vi "play-AFM-CS-imaging-dirty.vi"() -> ()   [LabVIEW 2017]
uses:
  raster-scan-params.ctl
  controls/PI-params.ctl
  controls/boolean_info.ctl
  <vilib>/userdefined/High Color/nirio_resource_hc.ctl
  <vilib>/Utility/file.llb/Read Delimited Spreadsheet (DBL).vi
  <vilib>/FPGAPlugInAG/cRIO-9082/niLvFpga_Open_cRIO-9082.vi
  <vilib>/rvi/interface/common/dynamic/niFpgaDynamicAddResources.vi
  <vilib>/FPGAPlugInAG/Dynamic/niLvFpga_Reset_Dynamic.vi
  <vilib>/rvi/interface/common/niFpgaWaitOnOcc.vi
  <vilib>/Utility/error.llb/Error Cluster From Error Code.vi
  <vilib>/rvi/errors/niLvFpgaAdjustHostInterfaceError.vi
  <vilib>/FPGAPlugInAG/Dynamic/niLvFpga_Run_Dynamic.vi
  <vilib>/Utility/file.llb/Write Delimited Spreadsheet (DBL).vi
  <vilib>/FPGAPlugInAG/Dynamic/niLvFpga_Close_Dynamic.vi
  <vilib>/rvi/interface/nirviOpenFPGA/nirviOpenFPGA.xnode
  FPGA Bitfiles/afmimagingcontro_FPGATargetSPARTA_cs-scanning_gCu814jKz54.lvbitx
  <vilib>/rvi/interface/nirviMethod/nirviMethod.xnode
  <vilib>/rvi/interface/nirviReadWriteControl/nirviReadWriteControl.xnode
  <vilib>/rvi/interface/nirviCloseFPGA/nirviCloseFPGA.xnode
  <vilib>/FPGAPlugInAG/Dynamic/niLvFpga_ConfigureFifo_Dynamic.vi
  <vilib>/rvi/errors/niLvFpgaMergeErrorWithErrorCode.vi
  <vilib>/rvi/interface/Simulation/niFpgaSimulationCallBeginRW.vi
  <vilib>/FPGAPlugInAG/Dynamic/niLvFpga_ReadFifo_Dynamic.vi
  NiFpgaLv.dll
  <vilib>/FPGAPlugInAG/Dynamic/niLvFpga_WriteFifo_Dynamic.vi
panel:
  in  "Z-settled-samples threshold":i16
  in  "Z-error-threshold":sgl
  out "case-selected":i16
  out "number-settled-samples-y":i16
  out "number-settled-samples-x":i16
  in  "settled-samples threshold":i16=200
  in  "error-threshold":sgl=0.1
  out "Array":i32[][](array[numeric])
  in  "zup-N":i16=5000
  out "z-control":dbl[](graph)
  out "x-axis 2":dbl[](graph)
  out "z-error":dbl[](graph)
  out "y-axis 2":dbl[](graph)
  out "size(s) 2":i32[](array[numeric])
  in  "numEntities":i16
  out "uz-":dbl[](graph)
  out "y-axis":dbl[](graph)
  out "x-axis":dbl[](graph)
  in  "z-bound":sgl=5.0
  in  "Ki-xy":sgl=0.005
  out "boolean errors":T1
  in  "raster-scan-params":T2={"TsTicks"=1600, "Stop"=TRUE, "TOL"=0.3, "ramp-rate"=-5e-06, "z-u-max"=5.0, "PI-params"={"Ki"=0.001, "setpoint"=0.0}} {"ramp-rate" format="%#_4g"; "TOL" format="%#_13g"}
  out "e(0) (threshhold init)":fxp<+/-,16,5>
  in  "STOP":bool
  out "nsamps":i32
  in  "trigger-0":bool
  in  "init Z up":sgl step=1
  in  "z_UP (case 3)":fxp<+/-,16,5>=1.0
  out "ADC-zaxis":sgl
  out "elements left":i32=1
  in  "reference traj path":path=path "C:/Users/arnold/Documents/labview/afm_imaging/data/data-in.csv"
  in  "outputData BOTH":path=path "C:/Users/arnold/Documents/labview/afm_imaging/data/data-out.csv"
  out "y iter":i32
  out "size(s)":i32
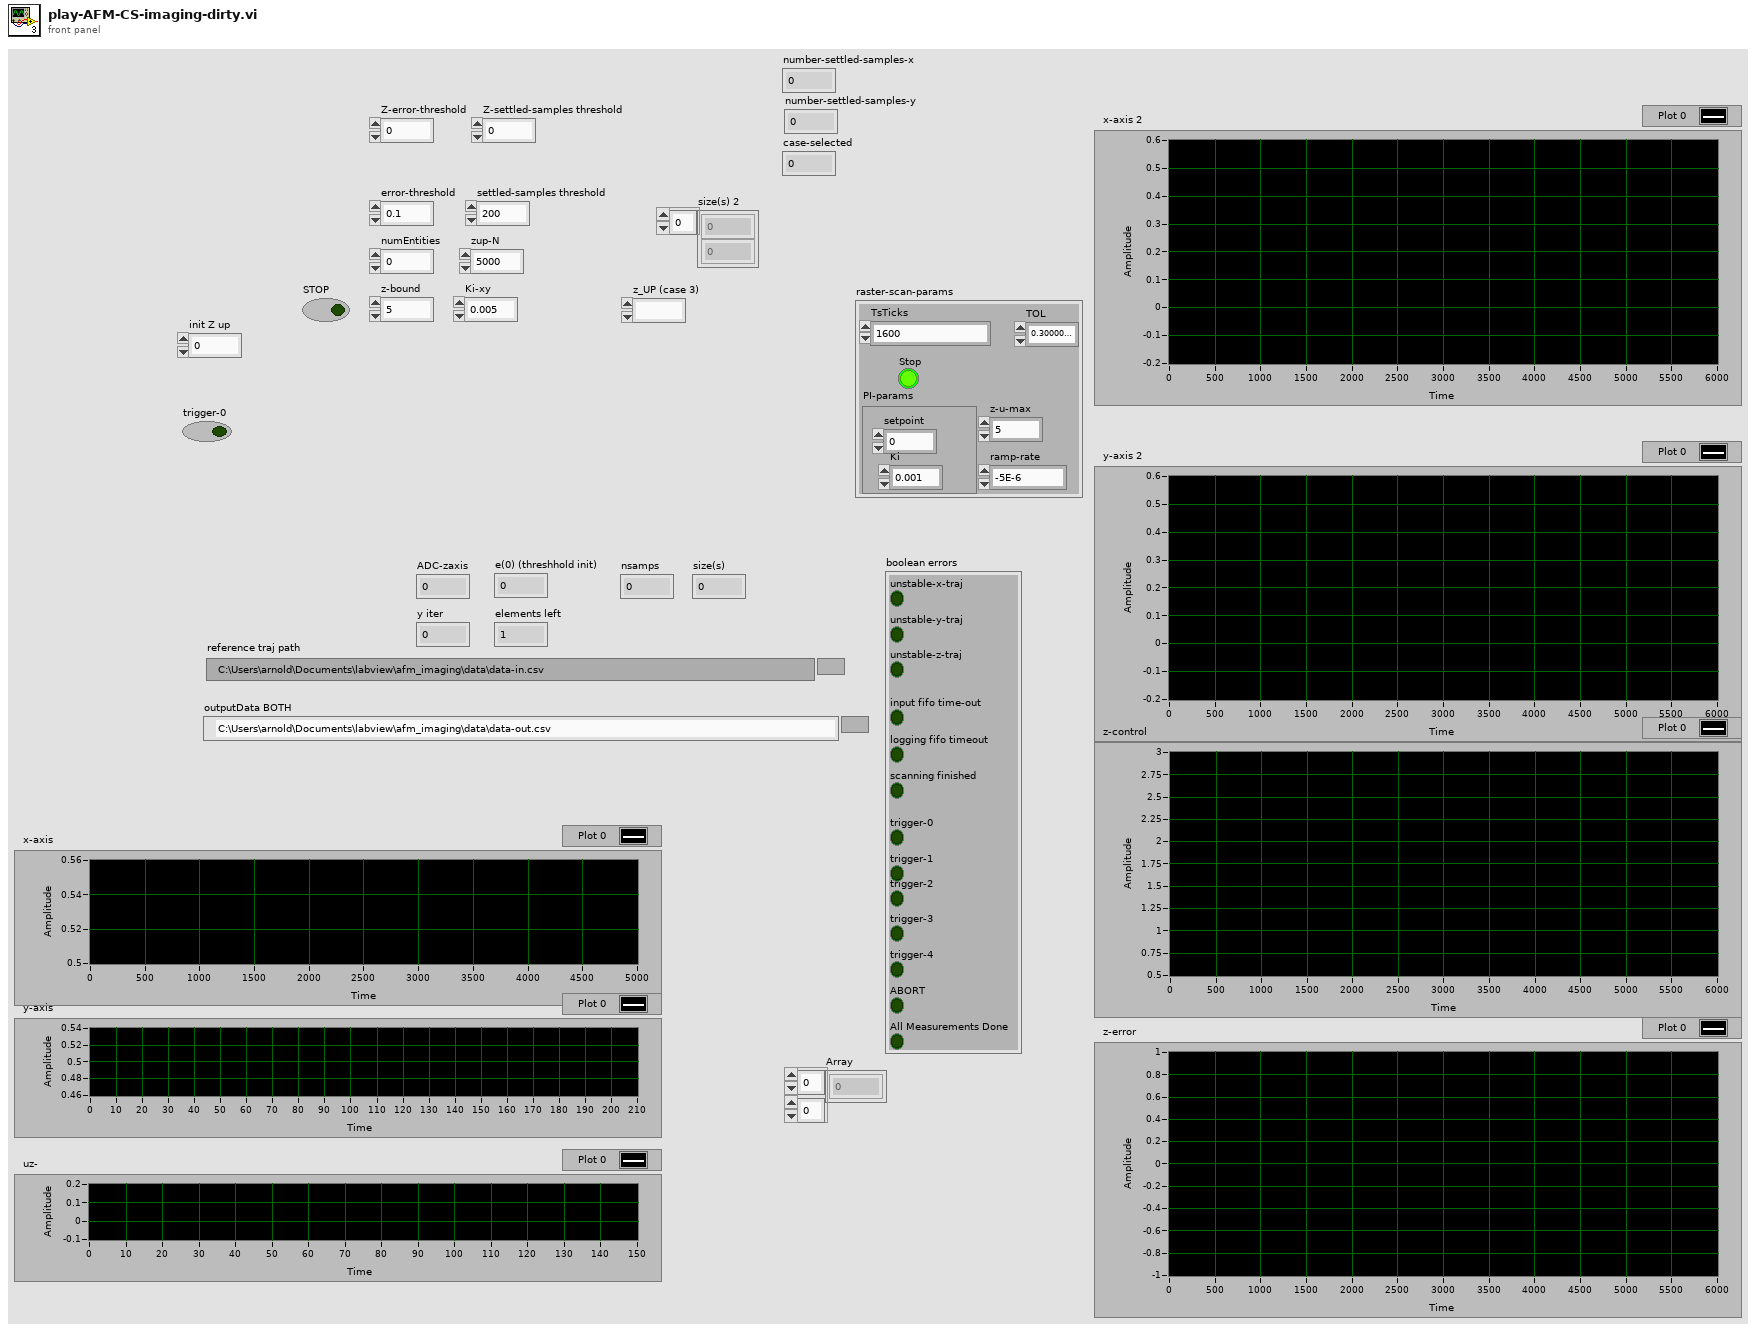
[diagram p1: front panel]
types:
  T1 = typedef "boolean_info.ctl" = cluster{"unstable-z-traj":bool, "input fifo time-out":bool, "logging fifo timeout":bool, "scanning finished":bool, "trigger-1":bool, "trigger-0":bool, "trigger-2":bool, "trigger-3":bool, "trigger-4":bool, "unstable-x-traj":bool, "unstable-y-traj":bool, "ABORT":bool, "All Measurements Done":bool}
  T2 = typedef "raster-scan-params.ctl" = cluster{"TsTicks":u32, "Stop":bool, "TOL":sgl, "ramp-rate":sgl, "z-u-max":sgl, "PI-params":T3}
  T3 = typedef "PI-params.ctl" = cluster{"Ki":sgl, "setpoint":sgl}
  T4 = typedef "nirio_resource_hc.ctl" = tag
  T5 = cluster{"unstable-z-traj":bool, "input fifo time-out":bool, "logging fifo timeout":bool, "scanning finished":bool, "trigger-1":bool, "trigger-0":bool, "trigger-2":bool, "trigger-3":bool, "trigger-4":bool, "unstable-x-traj":bool, "unstable-y-traj":bool, "ABORT":bool, "All Measurements Done":bool}
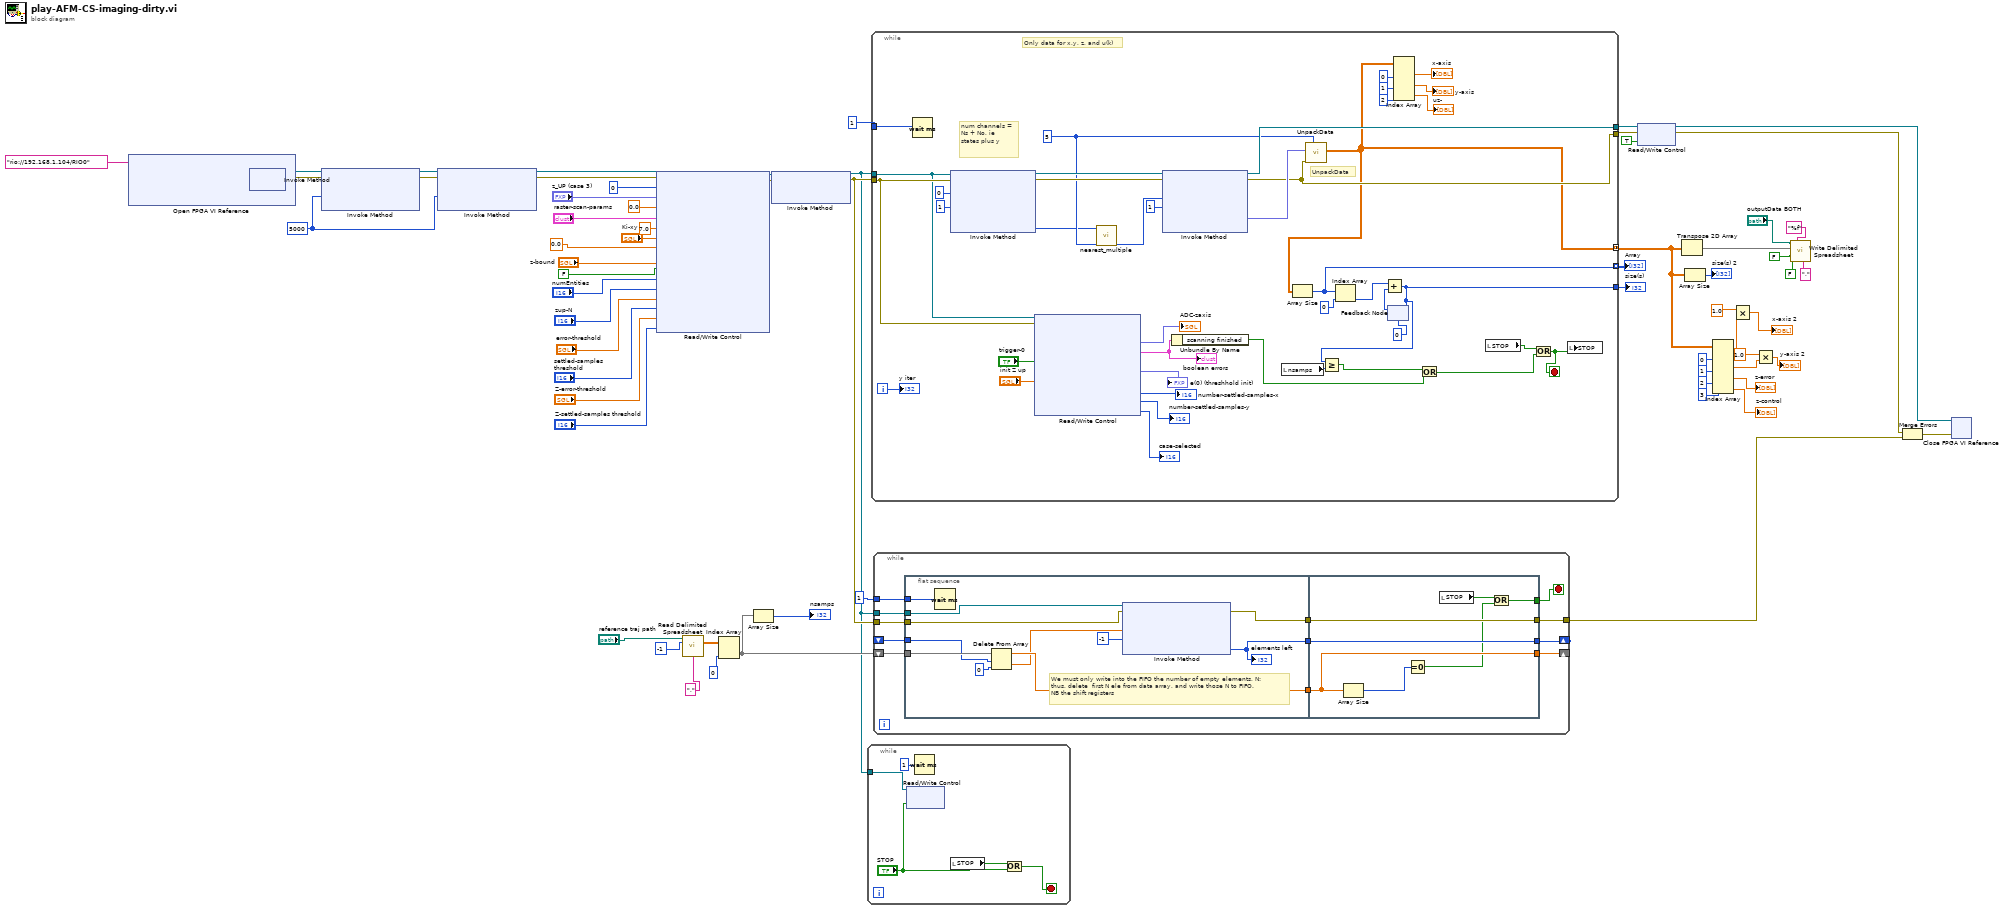
[diagram p0: block diagram]
diagram:
  w63 = 5000
  n1 = xnode "Open FPGA VI Reference"("resource name"=T4 "rio://192.168.1.104/RIO0") -> ("FPGA VI Reference Out"=w62:refnum<k20>, "error out"=w61:errorcluster)  [unwired: 1 in]
  n2 = xnode "Invoke Method"("FPGA VI Reference In"=w62, "error in"=w61) -> ("FPGA VI Reference Out"=w50:refnum<k20>, "error out"=w49:errorcluster)
  n3 = xnode "Invoke Method"("FPGA VI Reference In"=w50, "error in"=w49, "Requested Depth"=w63) -> ("FPGA VI Reference Out"=w54:refnum<k20>, "error out"=w55:errorcluster)  [unwired: 1 out]
  n4 = xnode "Invoke Method"("FPGA VI Reference In"=w54, "error in"=w55, "Requested Depth"=w63) -> ("FPGA VI Reference Out"=w65:refnum<k20>, "error out"=w64:errorcluster)  [unwired: 1 out]
  n5 = xnode "Read/Write Control"("FPGA VI Reference In"=w65, "error in"=w64, "initial case"=i16 0, "z_UP"="z_UP (case 3)", "u_z(0)"=sgl 0.0 ("u(0)"), "raster-scan-params"="raster-scan-params", "xy-bound"=sgl 7.0, "Ki-xy"="Ki-xy", "init Z up"=sgl 0.0 ("u(0)"), "z-bound"="z-bound", "trigger-0"=FALSE, "numEntities"="numEntities", "zup-N"="zup-N", "error-threshold"="error-threshold", "settled-samples threshold"="settled-samples threshold", "Z-error-threshold"="Z-error-threshold", "Z-settled-samples threshold"="Z-settled-samples threshold") -> ("FPGA VI Reference Out"=w52:refnum<k20>, "error out"=w51:errorcluster)
  n6 = call-poly <vilib>:"Read Delimited Spreadsheet.vi"("file path (dialog if empty)"="reference traj path", "number of rows (all:-1)"=-1, "delimiter (\\t)"=",") -> ("all rows"=w40:dbl[][])  [unwired: 7 in, 5 out]
  n7 = Index Array(array=w40, index (col)=0 ("dimension size")) -> (element=w47:dbl[])  [unwired: 1 in]
  n8 = Array Size(array=w47) -> (size(s)=→"nsamps":i32)
  n9 = xnode "Invoke Method"("FPGA VI Reference In"=w52, "error in"=w51) -> ("FPGA VI Reference Out"=w12:refnum<k20>, "error out"=w56:errorcluster)  [unwired: 1 in]
  n10 = while {
    tunnel: w12 -> [w72]
    stop <- w68 stop-if-true
    n11 = xnode "Read/Write Control"("FPGA VI Reference In"=w72, "ABORT"="STOP") -> ()  [unwired: 1 in, 2 out]
    n12 = Wait (ms)(milliseconds to wait=u32 1) -> ()  [unwired: 1 out]
    n13 = local read "STOP"() -> (w69:bool)
    n14 = Or(x=w69, y="STOP") -> (x .or. y?=w68:bool)
  }
  n15 = while {
    tunnel: 1 -> [w114]
    tunnel: w12 -> [w100]
    tunnel: w56 -> [w101]
    tunnel: [w107] -> w33
    tunnel: [w85] -> w16 mode=concatenating
    tunnel: [w98] -> w66
    tunnel: [w86] -> w32
    tunnel: [w76] -> w11 mode=indexing
    i -> [w99]
    stop <- w77 stop-if-true
    w91 = u32 5 ("y")
    # "num channels = Ns + No, ie states plus y"
    # "Only data for x,y, z, and u(k)"
    # "UnpackData"
    n16 = Wait (ms)(milliseconds to wait=w114) -> ()  [unwired: 1 out]
    n17 = xnode "Invoke Method"("FPGA VI Reference In"=w100, "error in"=w101, "Number of Elements"=0 ("Timeout (ms)"), "Timeout (ms)"=1) -> ("FPGA VI Reference Out"=w110:refnum<k20>, "error out"=w111:errorcluster, "Elements Remaining"=w90:u32)  [unwired: 1 out]
    n18 = xnode "Read/Write Control"("FPGA VI Reference In"=w100, "error in"=w101, "trigger-0"="trigger-0", "init Z up"="init Z up") -> ("ADC-zaxis"=→"ADC-zaxis":fxp<+/-,24,5>, "boolean indicators"=w88:T5, "e(0) (threshhold init)"=→"e(0) (threshhold init)":fxp<+/-,16,5>, "number-settled-samples-x"=→"number-settled-samples-x":i16, "number-settled-samples-y"=→"number-settled-samples-y":i16, "case-selected"=→"case-selected":i16)  [unwired: 1 in, 2 out]
    "boolean errors" <- w88
    n19 = call "nearest_multiple.vi"("numChan"=w91, "N"=w90) -> ("(int) y*floor(x/y)"=w89:u64)  [unwired: 9 in]
    n20 = xnode "Invoke Method"("FPGA VI Reference In"=w110, "error in"=w111, "Number of Elements"=w89, "Timeout (ms)"=1) -> ("FPGA VI Reference Out"=w107:refnum<k20>, "error out"=w86:errorcluster, "Data"=w105:fxp<+/-,16,5>[])  [unwired: 1 out]
    n21 = Unbundle By Name(w88) -> ("scanning finished"=w92:bool)
    n22 = local read "nsamps"() -> (w106:i32)
    n23 = call "UnpackData.vi"("NumChannels"=w91, "error In"=w86, "1D Data In"=w105) -> ("2D Data Out"=w85:dbl[][])  [unwired: 7 in, 1 out]
    n24 = Array Size(array=w85) -> (size(s)=w76:i32[])
    n25 = Index Array(array=w76, index=0) -> (element=w103:i32)
    n26 = feedback #1(0) -> (w104:i32)
    n27 = Add(x=w103, y=w104) -> (x+y=w98:i32)
    n28 = Greater Or Equal?(x=w98, y=w106) -> (x >= y?=w87:bool)
    n29 = feedback-in #1(w98) -> ()
    n30 = Index Array(array=w85, index (col) #1=0 ("disabled index (col)"), index (col) #2=1 ("index (col)"), index (col) #3=2 ("index (col)")) -> (element #1=→"x-axis":dbl[], element #2=→"y-axis":dbl[], element #3=→"uz-":dbl[])  [unwired: 3 in]
    n31 = Or(x=w87, y=w92) -> (x .or. y?=w96:bool)
    n32 = local read "STOP"() -> (w78:bool)
    n33 = Or(x=w78, y=w96) -> (x .or. y?=w77:bool)
    n34 = local write "STOP"(w77) -> ()
    "y iter" <- w99
  }
  "size(s)" <- w66
  "Array" <- w11
  n35 = while {
    tunnel: [w124] -> w53
    tunnel: 1 -> [w126]
    shift-right: [w120] -> _
    shift-left: _ -> [w123]
    shift-right: [w118] -> _
    shift-left: w47 -> [w125]
    tunnel: w12 -> [w117]
    tunnel: w56 -> [w116]
    stop <- w115 stop-if-true
    n36 = flat-sequence {
      tunnel: w126 -> [w137]
      tunnel: w125 -> [w132]
      tunnel: w123 -> [w128]
      tunnel: [w135] -> w122
      tunnel: [w133] -> w121
      tunnel: [w134] -> w119
      tunnel: w117 -> [w130]
      tunnel: w116 -> [w129]
      tunnel: [w144] -> w120
      tunnel: [w141] -> w124
      tunnel: w122 -> [w141]
      tunnel: w121 -> [w144]
      tunnel: w119 -> [w142]
      tunnel: [w142] -> w118
      tunnel: [w138] -> w115
      frame #0 {
        # "We must only write into the FIFO the number of empty elements, N:\nthus, delete  first N ele from data array, and write those N to FIFO.\nNB the shift registers"
        n37 = Wait (ms)(milliseconds to wait=w137) -> ()  [unwired: 1 out]
        n38 = Delete From Array(array=w132, length=w128, index=0) -> (deleted portion=w131:dbl[], array with subset deleted=w134:dbl[])
        n39 = xnode "Invoke Method"("FPGA VI Reference In"=w130, "error in"=w129, "Data"=w131, "Timeout (ms)"=-1) -> ("error out"=w135:errorcluster, "Empty Elements Remaining"=w133:u32)  [unwired: 1 out]
        "elements left" <- w133
      }
      frame #1 {
        n40 = Array Size(array=w142) -> (size(s)=w143:i32)
        n41 = Equal To 0?(x=w143) -> (x = 0?=w140:bool)
        n42 = local read "STOP"() -> (w139:bool)
        n43 = Or(x=w139, y=w140) -> (x .or. y?=w138:bool)
      }
    }
  }
  n44 = xnode "Read/Write Control"("FPGA VI Reference In"=w33, "error in"=w32, "ABORT"=TRUE) -> ("FPGA VI Reference Out"=w30:refnum<k20>, "error out"=w29:errorcluster)
  n45 = Transpose 2D Array(2D array=w16) -> (transposed array=w37:dbl[][])
  n46 = Array Size(array=w16) -> (size(s)=→"size(s) 2":i32[])
  n47 = Index Array(array=w16, index (col) #1=0 ("disabled index (col)"), index (col) #2=1 ("index (col)"), index (col) #3=2 ("index (col)"), index (col) #4=3 ("index (col)")) -> (element #1=w8:dbl[], element #2=w4:dbl[], element #3=→"z-error":dbl[], element #4=→"z-control":dbl[])  [unwired: 4 in]
  n48 = Multiply(x=1.0, y=w8) -> (x*y=→"x-axis 2":dbl[])
  n49 = Multiply(x=1.0, y=w4) -> (x*y=→"y-axis 2":dbl[])
  n50 = call-poly <vilib>:"Write Delimited Spreadsheet.vi"("file path (dialog if empty)"="outputData BOTH", "format (%.3f)"="%f", "2D data"=w37, "append to file? (new file:F)"=FALSE, "transpose? (no:F)"=FALSE, "delimiter (\\t)"=",") -> ()  [unwired: 8 in, 2 out]
  n51 = Merge Errors(w29, w53) -> (w57:errorcluster)
  n52 = xnode "Close FPGA VI Reference"("FPGA VI Reference In"=w30, "error in"=w57) -> ()  [unwired: 1 out]
